vi "Read PS3 control.vi"(8 "error in (no error)":errorcluster, 11 "Controller Reference In":refnum<k1>) -> (0 "error out":errorcluster, 2 "PS3 Controls":T1 {"Left Analogue Stick X" scale=-32768.0..32768.0; "Left Analogue Stick Y" scale=32768.0..-32768.0; "Right Analogue Stick X" scale=-32768.0..32768.0; "Right Analogue Stick Y" scale=32768.0..-32768.0; "X Rotation" scale=-32768.0..32768.0; "Y Rotation" scale=-32768.0..32768.0; "L2 Pressure" scale=0.0..32768.0; "Numeric" format="%d°"}, 3 "Controller Reference Out":refnum<k1>)   [LabVIEW 2024]
doc: "This VI takes in the information from Windows and the MotioninJoy driver."
uses:
  Controls/PS3 Controls.ctl
  <vilib>/Utility/inputDevices.llb/joystickAcquire.vi
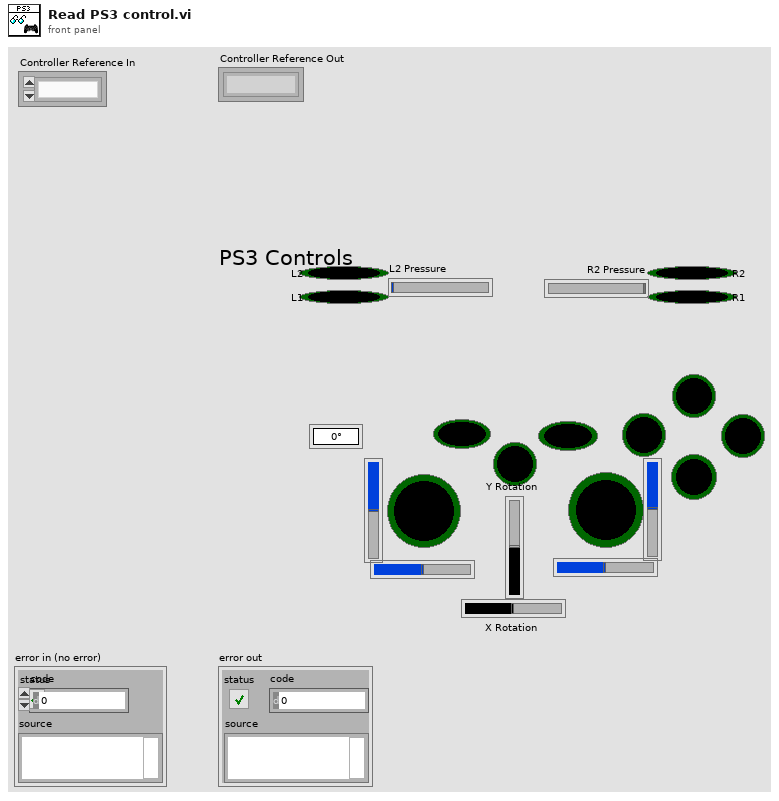
[diagram p1: front panel]
types:
  T1 = typedef "PS3 Controls.ctl" = cluster{"Left Analogue Stick X":i32, "Left Analogue Stick Y":i32, "Right Analogue Stick X":i32, "Right Analogue Stick Y":i32, "Y Rotation":i32, "X Rotation":i32, "L2 Pressure":i32, "R2 Pressure":i32, "Triangle":bool, "Circle":bool, "X":bool, "Square":bool, "L1":bool, "R1":bool, "L2":bool, "R2":bool, "L3":bool, "R3":bool, "Select":bool, "Start":bool, "PS Button":bool, "Numeric":i32}
  T2 = cluster{"X axis":i32, "Y axis":i32, "Z axis":i32, "X axis rotation":i32, "Y axis rotation":i32, "Z axis rotation":i32, "U axis":i32, "V axis":i32}
  T3 = cluster{"button 1":bool, "button 2":bool, "button 3":bool, "button 4":bool, "button 5":bool, "button 6":bool, "button 7":bool, "button 8":bool, "button 9":bool, "button 10":bool, "button 11":bool, "button 12":bool, "button 13":bool, "button 14":bool, "button 15":bool, "button 16":bool, "button 17":bool, "button 18":bool, "button 19":bool, "button 20":bool, "button 21":bool, "button 22":bool, "button 23":bool, "button 24":bool, "button 25":bool, "button 26":bool, "button 27":bool, "button 28":bool, "button 29":bool, "button 30":bool, "button 31":bool, "button 32":bool}
  T4 = cluster{"pov 1":i32, "pov 2":i32, "pov 3":i32, "pov 4":i32}
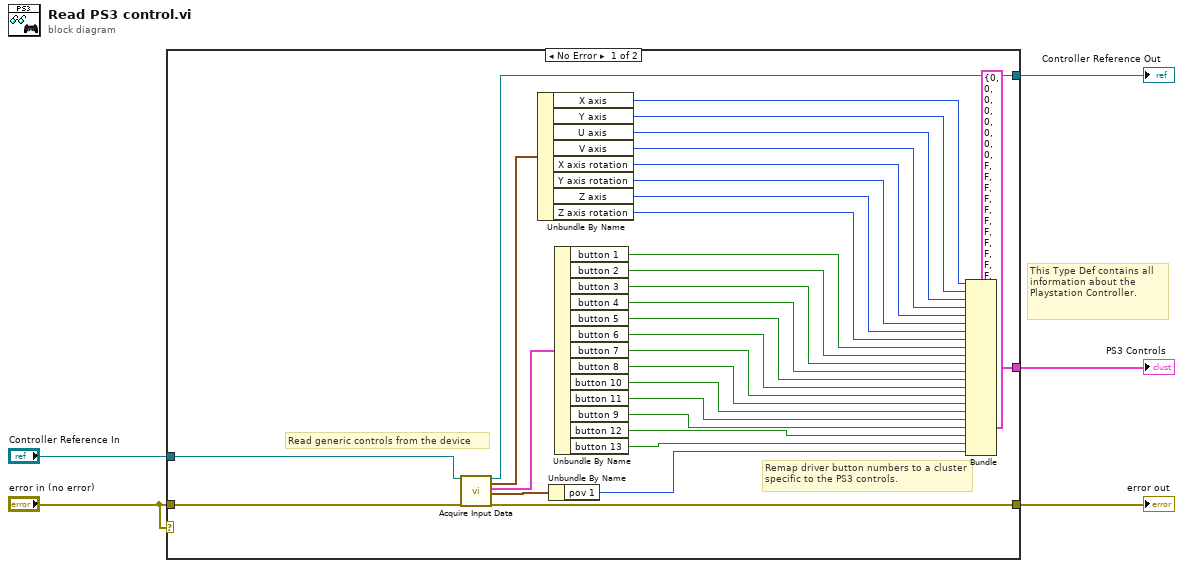
[diagram p0: block diagram]
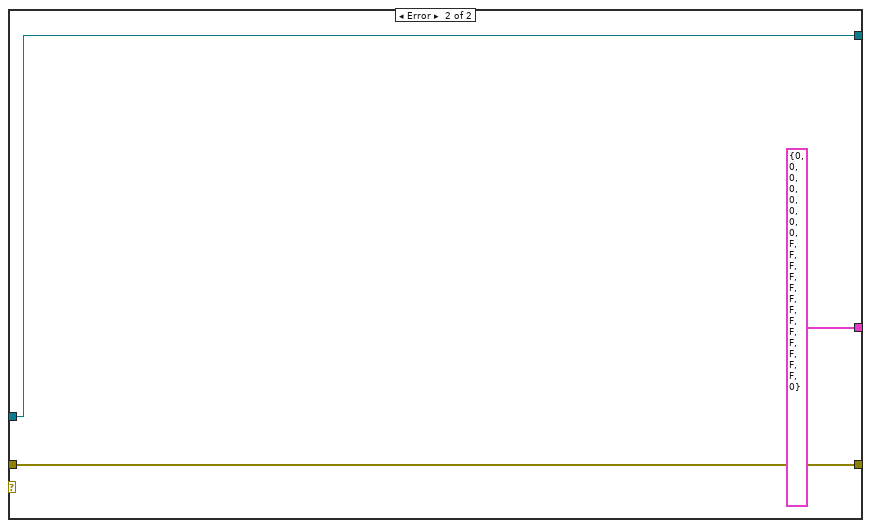
[diagram p2: hidden frame]
diagram:
  # "This Type Def contains all information about the Playstation Controller."
  n1 = case shown="No Error" "error in (no error)" {
    tunnel: "Controller Reference In" -> [w11 w39]
    tunnel: "error in (no error)" -> [w10 w37]
    tunnel: [w8 T1 {"Left Analogue Stick X"=0, "Left Analogue Stick Y"=0, "Right Analogue Stick X"=0, "Right Analogue Stick Y"=0, "Y Rotation"=0, "X Rotation"=0, "L2 Pressure"=0, "R2 Pressure"=0, "Triangle"=FALSE, "Circle"=FALSE, "X"=FALSE, "Square"=FALSE, "L1"=FALSE, "R1"=FALSE, "L2"=FALSE, "R2"=FALSE, "L3"=FALSE, "R3"=FALSE, "Select"=FALSE, "Start"=FALSE, "PS Button"=FALSE, "Numeric"=0} ("PS3 Controls")] -> w4
    tunnel: [w7 w39] -> w3
    tunnel: [w6 w37] -> w1
    frame No Error {
      # "Read generic controls from the device"
      # "Remap driver button numbers to a cluster specific to the PS3 controls."
      n2 = call-poly <vilib>:"Acquire Input Data.vi"("device ID"=w11, "error in (no error)"=w10) -> ("device ID"=w7:refnum<k1>, "axis info"=w12:T2, "button info"=w13:T3, "direction info"=w14:T4, "error out"=w6:errorcluster)  [unwired: 13 out]
      n3 = Unbundle By Name(w12) -> ("X axis"=w23:i32, "Y axis"=w24:i32, "U axis"=w25:i32, "V axis"=w26:i32, "X axis rotation"=w27:i32, "Y axis rotation"=w28:i32, "Z axis"=w29:i32, "Z axis rotation"=w30:i32)
      n4 = Unbundle By Name(w14) -> ("pov 1"=w22:i32)
      n5 = Unbundle By Name(w13) -> ("button 1"=w15:bool, "button 2"=w16:bool, "button 3"=w17:bool, "button 4"=w18:bool, "button 5"=w19:bool, "button 6"=w20:bool, "button 7"=w21:bool, "button 8"=w31:bool, "button 10"=w32:bool, "button 11"=w33:bool, "button 9"=w34:bool, "button 12"=w35:bool, "button 13"=w36:bool)
      n6 = Bundle(cluster=T1 {"Left Analogue Stick X"=0, "Left Analogue Stick Y"=0, "Right Analogue Stick X"=0, "Right Analogue Stick Y"=0, "Y Rotation"=0, "X Rotation"=0, "L2 Pressure"=0, "R2 Pressure"=0, "Triangle"=FALSE, "Circle"=FALSE, "X"=FALSE, "Square"=FALSE, "L1"=FALSE, "R1"=FALSE, "L2"=FALSE, "R2"=FALSE, "L3"=FALSE, "R3"=FALSE, "Select"=FALSE, "Start"=FALSE, "PS Button"=FALSE, "Numeric"=0} ("PS3 Controls"), "Left Analogue Stick X"=w23, "Left Analogue Stick Y"=w24, "Right Analogue Stick X"=w25, "Right Analogue Stick Y"=w26, "Y Rotation"=w27, "X Rotation"=w28, "L2 Pressure"=w29, "R2 Pressure"=w30, "Triangle"=w15, "Circle"=w16, "X"=w17, "Square"=w18, "L1"=w19, "R1"=w20, "L2"=w21, "R2"=w31, "L3"=w32, "R3"=w33, "Select"=w34, "Start"=w35, "PS Button"=w36, "Numeric"=w22) -> (w8:T1)
    }
    frame Error {
    }
  }
  "PS3 Controls" <- w4
  "Controller Reference Out" <- w3
  "error out" <- w1
